vi "st_eval CDF (student).vi"(4 "parameters":variant, 5 "x":dbl) -> (2 "f(x)":dbl)   [LabVIEW 2020, in "NI_Gmath.lvlib"]
uses:
  <vilib>/gmath/NI_Gmath.lvlib
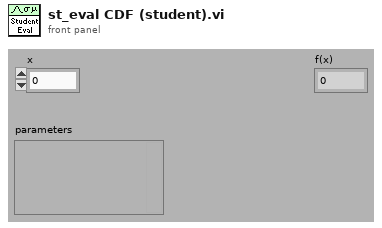
[diagram p1: front panel]
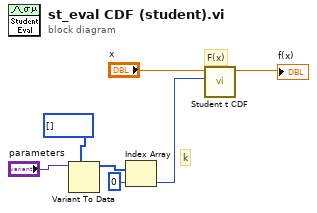
[diagram p0: block diagram]
diagram:
  # "k"
  # "F(x)"
  n1 = Variant To Data(type=i32[] [], Variant="parameters") -> (data=w5:i32[])  [unwired: 1 in, 1 out]
  n2 = Index Array(array=w5, index=0) -> (element=w3:i32)
  n3 = call <vilib>:"Student t CDF.vi"("k degrees of freedom"=w3, "x"="x") -> ("cdf(x)"=→"f(x)":dbl)  [unwired: 7 in, 2 out]
